vi "test-Function-Generator-Test1.vi"(8 "error in (no error)":errorcluster) -> (0 "error out":errorcluster, 3 "All tests passed":bool)   [LabVIEW 2019]
uses:
  <vilib>/Rock Robotics/WPI/ThirdParty/JAS_Junk/TrajLib/X_Y_PAIR.ctl
  <vilib>/Rock Robotics/WPI/ThirdParty/JAS_Junk/TrajLib/FunctionGenerator_Add_Value.vi
  <vilib>/gmath/interp.llb/Search Ordered Table.vi
  <vilib>/Rock Robotics/WPI/ThirdParty/JAS_Junk/TrajLib/Trajectory_Library.lvlib
panel:
  out "Output T 8":dbl
  out "Output T 7":dbl
  out "Output T 6":dbl
  out "Output T 5":dbl
  out "Output T 4":dbl
  out "Output T 3":dbl
  out "Table Ys":dbl[](array[numeric])
  out "Table Xs":dbl[](array[numeric])
  out "Output T 2":dbl
  out "Output T 1":dbl
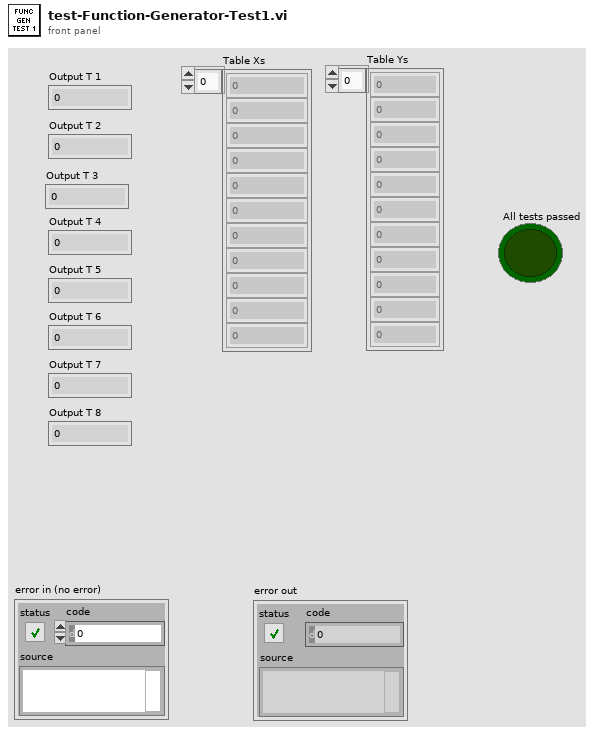
[diagram p1: front panel]
types:
  T1 = typedef "Trajectory_Library.lvlib/X_Y_PAIR.ctl" = cluster{"X":dbl, "Y":dbl}
  T2 = typedef "Trajectory_Library.lvlib/FUNCTION_GENERATOR.ctl" = cluster{"Table Xs":dbl[], "Table Ys":dbl[], "MinX":dbl, "MaxX":dbl, "ItemCount":i32}
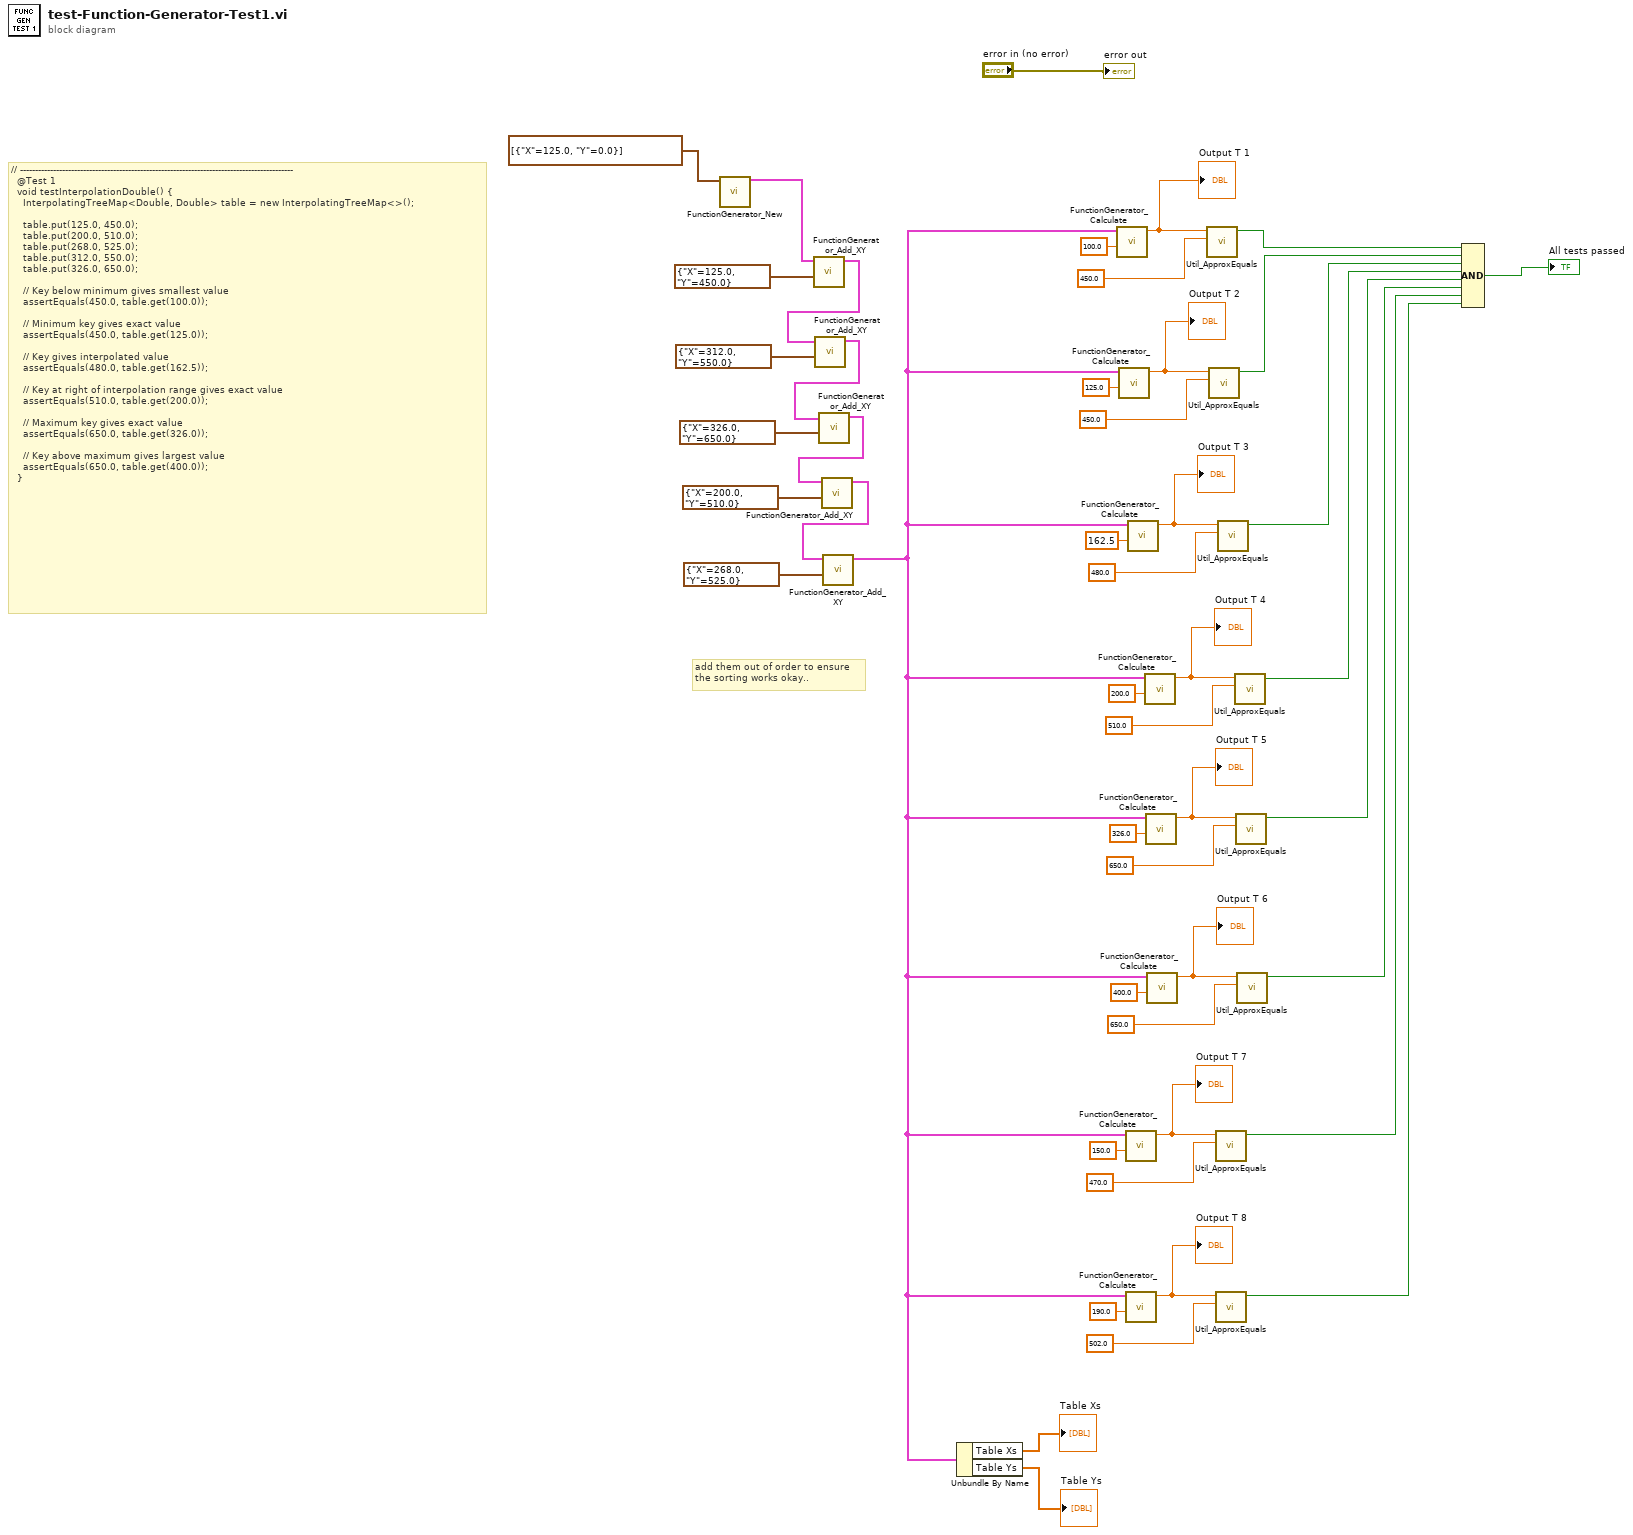
[diagram p0: block diagram]
diagram:
  # "add them out of order to ensure\nthe sorting works okay.."
  # "// -------------------------------------------------------------------------------------------\n  @Test 1\n  void testInterpolationDouble() {\n    InterpolatingTreeMap<Double, Double> table = new InterpolatingTreeMap<>();\n\n    table.put(125.0, 450.0);\n    table.put(200.0, 510.0);\n    table.put(268.0, 525.0);\n    table.put(312.0, 550.0);\n    table.put(326.0, 650.0);\n\n    // Key below minimum gives smallest value\n    assertEquals(450.0, table.get(100.0));\n\n    // Minimum key gives exact value\n    assertEquals(450.0, table.get(125.0));\n\n    // Key gives interpolated value\n    assertEquals(480.0, table.get(162.5));\n\n    // Key at right of interpolation range gives exact value\n    assertEquals(510.0, table.get(200.0));\n\n    // Maximum key gives exact value\n    assertEquals(650.0, table.get(326.0));\n\n    // Key above maximum gives largest value\n    assertEquals(650.0, table.get(400.0));\n  }"
  n1 = call <vilib>:"FunctionGenerator_New.vi"("X Y Pairs"=T1[] [{"X"=125.0, "Y"=0.0}]) -> ("FUNCTION_GENERATOR"=w26:T2)  [unwired: 10 in]
  n2 = call <vilib>:"FunctionGenerator_Add_XY.vi"("X_Y_PAIR"=T1 {"X"=125.0, "Y"=450.0}, "in FUNCTION_GENERATOR"=w26) -> ("out FUNCTION_GENERATOR"=w41:T2)  [unwired: 9 in]
  n3 = call <vilib>:"FunctionGenerator_Add_XY.vi"("X_Y_PAIR"=T1 {"X"=312.0, "Y"=550.0}, "in FUNCTION_GENERATOR"=w41) -> ("out FUNCTION_GENERATOR"=w40:T2)  [unwired: 9 in]
  n4 = call <vilib>:"FunctionGenerator_Add_XY.vi"("X_Y_PAIR"=T1 {"X"=326.0, "Y"=650.0}, "in FUNCTION_GENERATOR"=w40) -> ("out FUNCTION_GENERATOR"=w39:T2)  [unwired: 9 in]
  n5 = call <vilib>:"FunctionGenerator_Add_XY.vi"("X_Y_PAIR"=T1 {"X"=200.0, "Y"=510.0}, "in FUNCTION_GENERATOR"=w39) -> ("out FUNCTION_GENERATOR"=w38:T2)  [unwired: 9 in]
  n6 = call <vilib>:"FunctionGenerator_Add_XY.vi"("X_Y_PAIR"=T1 {"X"=268.0, "Y"=525.0}, "in FUNCTION_GENERATOR"=w38) -> ("out FUNCTION_GENERATOR"=w3:T2)  [unwired: 9 in]
  n7 = Unbundle By Name(w3) -> ("Table Xs"=→"Table Xs":dbl[], "Table Ys"=→"Table Ys":dbl[])
  n8 = call <vilib>:"FunctionGenerator_Calculate.vi"("Input Value"=100.0, "FUNCTION_GENERATOR"=w3) -> ("Output Value"=w36:dbl)  [unwired: 9 in]
  "Output T 1" <- w36
  n9 = call <vilib>:"FunctionGenerator_Calculate.vi"("Input Value"=125.0, "FUNCTION_GENERATOR"=w3) -> ("Output Value"=w29:dbl)  [unwired: 9 in]
  "Output T 2" <- w29
  n10 = call <vilib>:"FunctionGenerator_Calculate.vi"("Input Value"=150.0, "FUNCTION_GENERATOR"=w3) -> ("Output Value"=w8:dbl)  [unwired: 9 in]
  "Output T 7" <- w8
  n11 = call <vilib>:"FunctionGenerator_Calculate.vi"("Input Value"=190.0, "FUNCTION_GENERATOR"=w3) -> ("Output Value"=w5:dbl)  [unwired: 9 in]
  "Output T 8" <- w5
  n12 = call <vilib>:"FunctionGenerator_Calculate.vi"("Input Value"=162.5, "FUNCTION_GENERATOR"=w3) -> ("Output Value"=w23:dbl)  [unwired: 9 in]
  "Output T 3" <- w23
  n13 = call <vilib>:"FunctionGenerator_Calculate.vi"("Input Value"=200.0, "FUNCTION_GENERATOR"=w3) -> ("Output Value"=w20:dbl)  [unwired: 9 in]
  "Output T 4" <- w20
  n14 = call <vilib>:"FunctionGenerator_Calculate.vi"("Input Value"=326.0, "FUNCTION_GENERATOR"=w3) -> ("Output Value"=w15:dbl)  [unwired: 9 in]
  "Output T 5" <- w15
  n15 = call <vilib>:"FunctionGenerator_Calculate.vi"("Input Value"=400.0, "FUNCTION_GENERATOR"=w3) -> ("Output Value"=w12:dbl)  [unwired: 9 in]
  "Output T 6" <- w12
  n16 = call <vilib>:"Util_ApproxEquals.vi"("Value 2"=450.0, "Value 1"=w36) -> ("ApproxEquals"=w34:bool)  [unwired: 9 in]
  n17 = call <vilib>:"Util_ApproxEquals.vi"("Value 2"=450.0, "Value 1"=w29) -> ("ApproxEquals"=w30:bool)  [unwired: 9 in]
  n18 = call <vilib>:"Util_ApproxEquals.vi"("Value 2"=470.0, "Value 1"=w8) -> ("ApproxEquals"=w2:bool)  [unwired: 9 in]
  n19 = call <vilib>:"Util_ApproxEquals.vi"("Value 2"=502.0, "Value 1"=w5) -> ("ApproxEquals"=w1:bool)  [unwired: 9 in]
  n20 = call <vilib>:"Util_ApproxEquals.vi"("Value 2"=480.0, "Value 1"=w23) -> ("ApproxEquals"=w19:bool)  [unwired: 9 in]
  n21 = call <vilib>:"Util_ApproxEquals.vi"("Value 2"=510.0, "Value 1"=w20) -> ("ApproxEquals"=w18:bool)  [unwired: 9 in]
  n22 = call <vilib>:"Util_ApproxEquals.vi"("Value 2"=650.0, "Value 1"=w15) -> ("ApproxEquals"=w11:bool)  [unwired: 9 in]
  n23 = call <vilib>:"Util_ApproxEquals.vi"("Value 2"=650.0, "Value 1"=w12) -> ("ApproxEquals"=w10:bool)  [unwired: 9 in]
  n24 = Compound Arithmetic op=AND(w34, w30, w19, w18, w11, w10, w2, w1) -> (→"All tests passed":bool)
  "error out" <- "error in (no error)"
